vi "solar_app SOLARini Read (STR).vi"(4 "Add Quotes? (T)":bool=TRUE, 5 "Write If Not Found? (T)":bool=TRUE, 6 "Comment (Create only)":string, 7 "Section (\"\"=solar)":string, 9 "Default Value (STR)":string, 10 "Key":string) -> (1 "Value (STR) out":string, 2 "Found?":bool)   [LabVIEW 2018]
doc: "This reads a string configuration key from the solar.ini configuration file."
uses:
  cfg/solar_cfg Read File (Str).vi
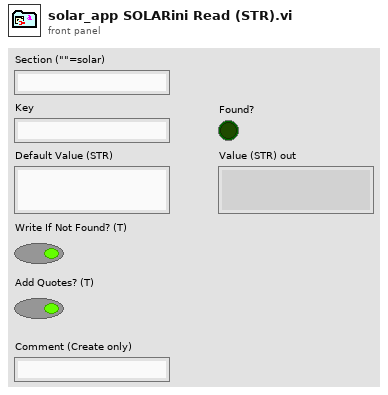
[diagram p1: front panel]
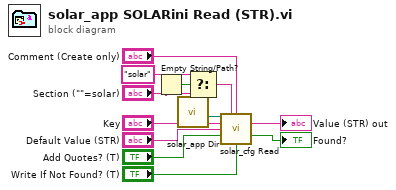
[diagram p0: block diagram]
diagram:
  n1 = Empty String/Path?(string/path="Section (\"\"=solar)") -> (empty?=w11:bool)
  n2 = call "solar_app Dir.vi"() -> ("solar.ini"=w12:path)  [unwired: 9 in, 2 out]
  n3 = Select(t="solar" ("Section (\"\" = Use Filename)"), s=w11, f="Section (\"\"=solar)") -> (s? t:f=w8:string)
  n4 = call-poly "solar_cfg Read.vi"("Config Path (*.ini)"=w12, "Section (\"\" = Use Filename)"=w8, "Comment"="Comment (Create only)", "Key"="Key", "Value in"="Default Value (STR)", "Add Quotes? (T)"="Add Quotes? (T)", "Write If Not Found? (T)"="Write If Not Found? (T)") -> ("Value out"=→"Value (STR) out":string, "Found?"=→"Found?":bool)  [unwired: 5 in, 2 out]
